vi "GetSystemInfoNames.vi"() -> (3 "Pos Info":T1)   [LabVIEW 2015]
uses:
  W:/GSCS/Systems/Coll_Focus/GSP_COLL_Global.vi
  W:/GSCS/Systems/Grating_Translation/GSP_GT_Global.vi
  W:/GSCS/Systems/Primary Filter/GSP_F1_Global.vi
  W:/GSCS/Systems/Secondary Filter/GSP_F2_Global.vi
  W:/GSCS/Systems/Slit/GSP_SLIT_Global.vi
  W:/GSCS/Systems/Wavelength/GSP_Wavelength_Global.vi
  W:/GSCS/Systems/Cam_Focus/GSP_CF_Global.vi
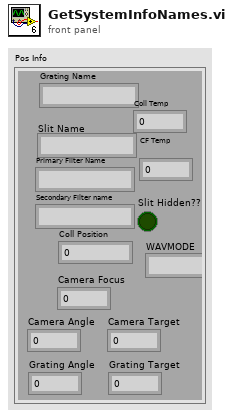
[diagram p1: front panel]
types:
  T1 = cluster{"Grating Name":string, "Slit Name":string, "Primary Filter Name":string, "Secondary Filter name":string, "Coll Position":i32, "Camera Focus":i32, "Camera Angle":dbl, "Grating Angle":dbl, "Coll Temp":dbl, "CF Temp\n":dbl, "Camera Target":dbl, "Grating Target":dbl, "WAVMODE":string, "Slit Hidden??":bool}
  T2 = cluster{"Grating Name":string, "Slit Name":string, "Primary Filter Name":string, "Secondary Filter Name":string, "Coll Position":i32, "Camera Focus":i32, "Camera Angle":dbl, "Grating Angle":dbl, "Coll Temp":dbl, "CF Temp":dbl, "Camera Target":dbl, "Grating Target":dbl, "WAVMODE":string, "Slit Hidden?":bool}
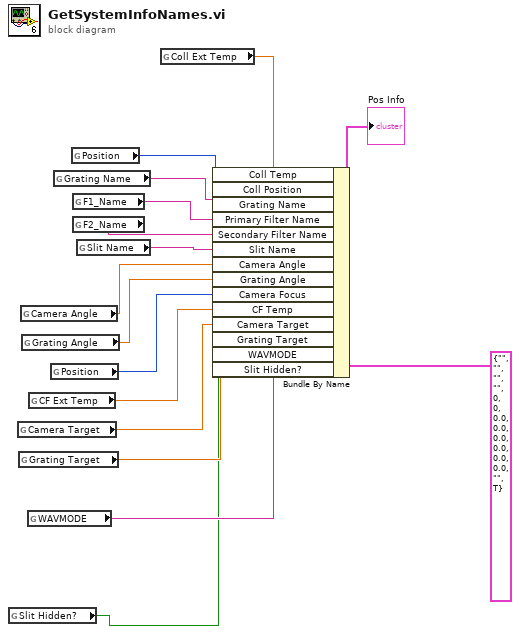
[diagram p0: block diagram]
diagram:
  n1 = global read "GSP_SLIT_Global.vi" "Slit Hidden?"() -> (w1:bool)
  n2 = global read "GSP_Wavelength_Global.vi" "Camera Target"() -> (w4:dbl)
  n3 = global read "GSP_Wavelength_Global.vi" "Grating Target"() -> (w3:dbl)
  n4 = global read "GSP_Wavelength_Global.vi" "Camera Angle"() -> (w11:dbl)
  n5 = global read "GSP_Wavelength_Global.vi" "Grating Angle"() -> (w10:dbl)
  n6 = global read "GSP_Wavelength_Global.vi" "WAVMODE"() -> (w2:string)
  n7 = global read "GSP_CF_Global.vi" "CF Ext Temp"() -> (w6:dbl)
  n8 = global read "GSP_CF_Global.vi" "Position"() -> (w9:i32)
  n9 = global read "GSP_GT_Global.vi" "Grating Name"() -> (w12:string)
  n10 = global read "GSP_COLL_Global.vi" "Position"() -> (w16:i32)
  n11 = global read "GSP_F1_Global.vi" "F1_Name"() -> (w15:string)
  n12 = global read "GSP_F2_Global.vi" "F2_Name"() -> (w14:string)
  n13 = global read "GSP_SLIT_Global.vi" "Slit Name"() -> (w13:string)
  n14 = global read "GSP_SLIT_Global.vi" "Coll Ext Temp"() -> (w5:dbl)
  n15 = Bundle By Name(cluster=T2 {"Grating Name"="", "Slit Name"="", "Primary Filter Name"="", "Secondary Filter Name"="", "Coll Position"=0, "Camera Focus"=0, "Camera Angle"=0.0, "Grating Angle"=0.0, "Coll Temp"=0.0, "CF Temp"=0.0, "Camera Target"=0.0, "Grating Target"=0.0, "WAVMODE"="", "Slit Hidden?"=TRUE} ("Pos Info"), "Coll Temp"=w5, "Coll Position"=w16, "Grating Name"=w12, "Primary Filter Name"=w15, "Secondary Filter Name"=w14, "Slit Name"=w13, "Camera Angle"=w11, "Grating Angle"=w10, "Camera Focus"=w9, "CF Temp"=w6, "Camera Target"=w4, "Grating Target"=w3, "WAVMODE"=w2, "Slit Hidden?"=w1) -> (→"Pos Info":T2)
